vi "MakeInitialOMFJSON.vi"(0 "OMF Container ID":string, 1 "OMF Static Type ID":string, 2 "OMF Static Type Property Names, Formats, and Values":T2(array[cluster]), 3 "OMF Dynamic Type ID":string, 4 "OMF Dynamic Type Property Names and Formats":T1(array[cluster]), 5 "OMF Static Type Instance Name":string) -> (14 "OMF Static Type Message JSON":string, 15 "OMF Dynamic Type Message JSON":string, 16 "OMF Container Message JSON":string, 17 "OMF Static Type Instance Message JSON":string, 18 "OMF Link Message JSON":string)   [LabVIEW 2014]
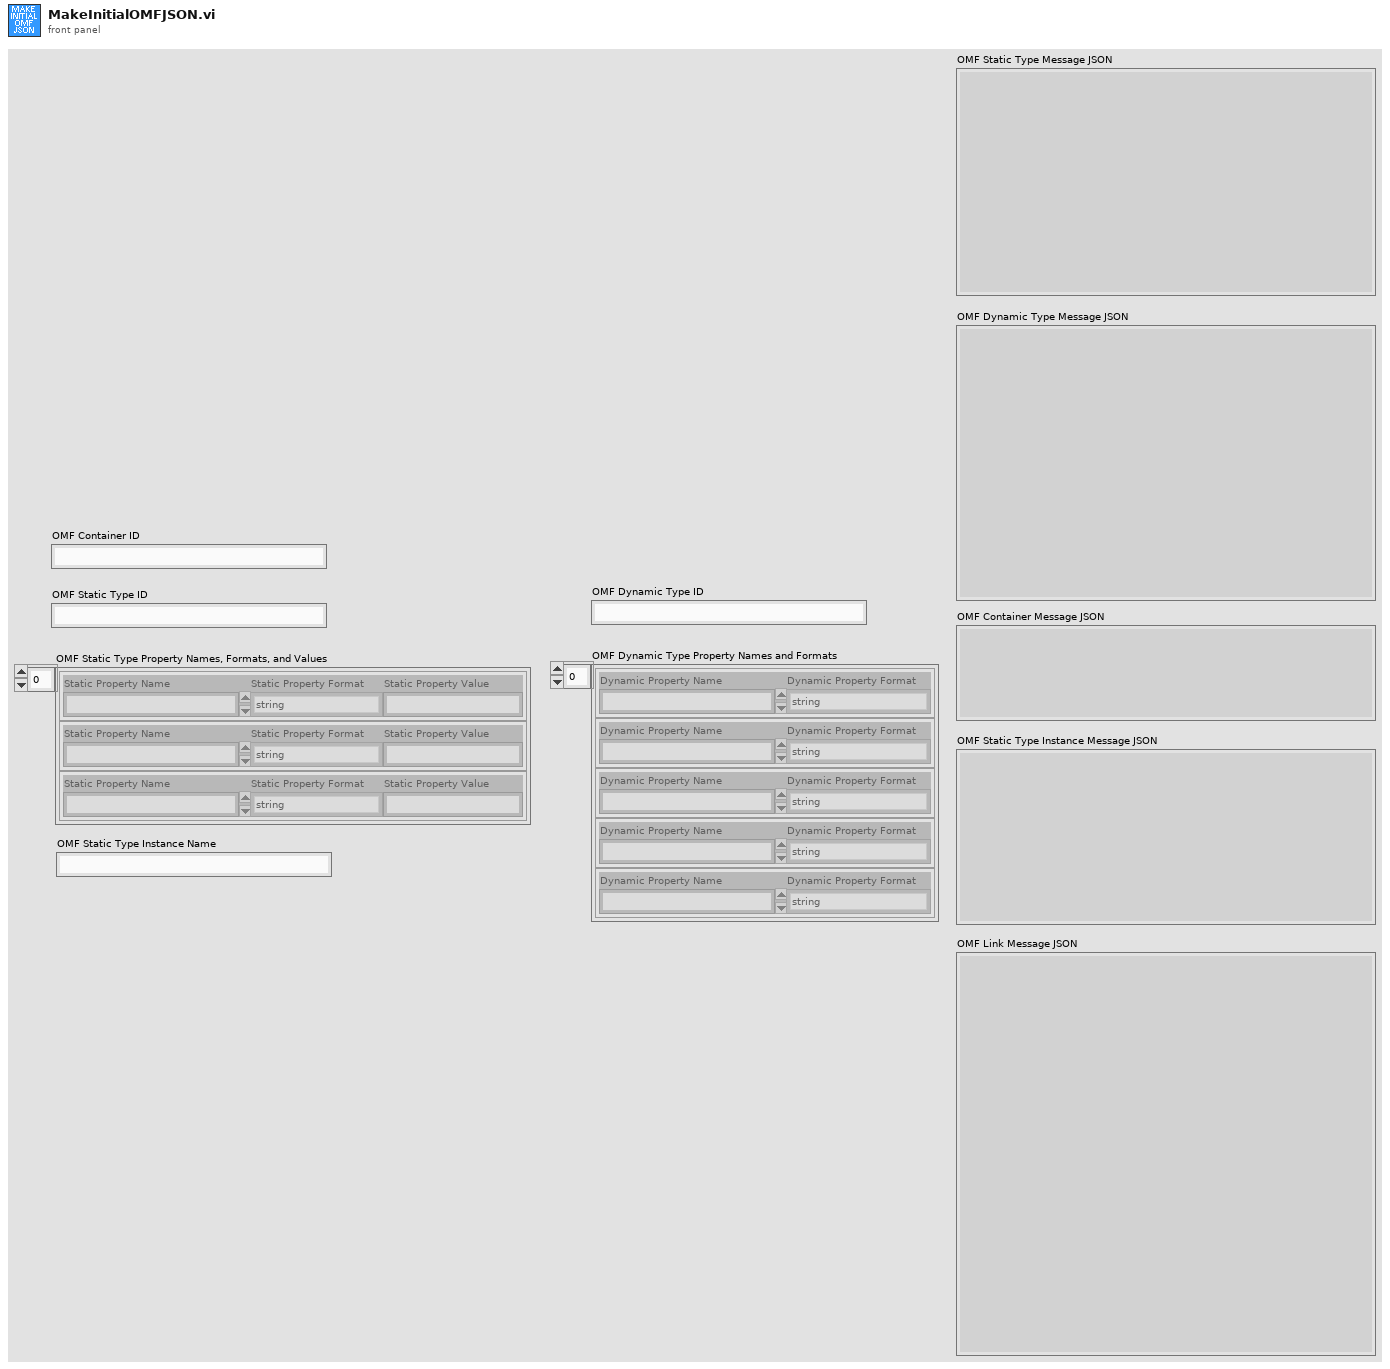
[diagram p1: front panel]
types:
  T1 = cluster{"Dynamic Property Name":string, "Dynamic Property Format":enum16{"string", "number"}}[]
  T2 = cluster{"Static Property Name":string, "Static Property Format":enum16{"string", "number"}, "Static Property Value":string}[]
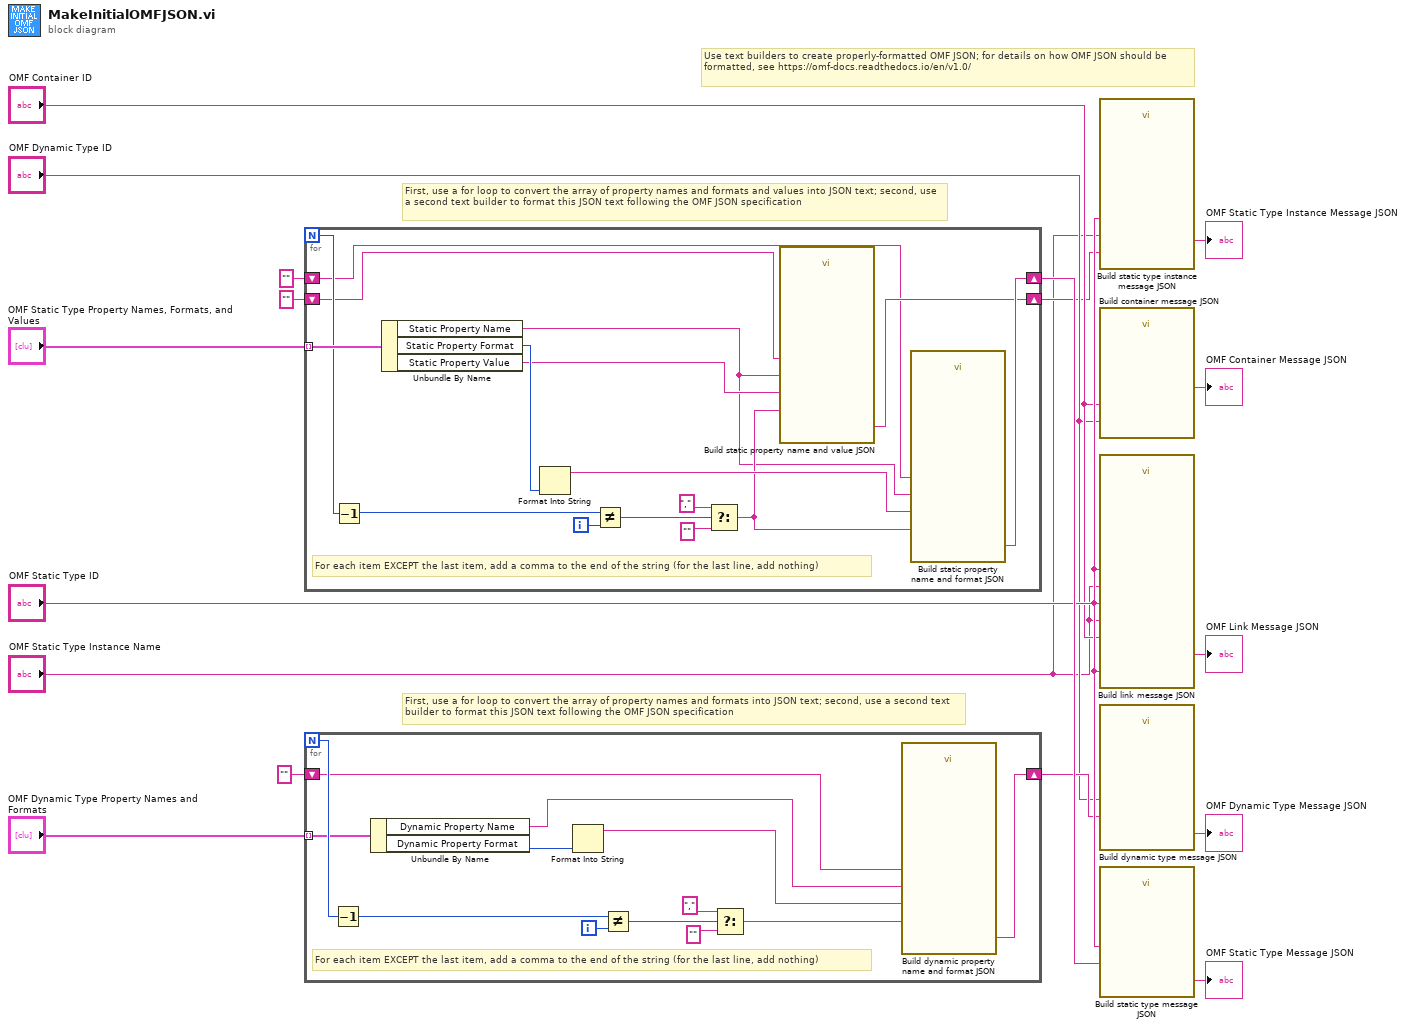
[diagram p0: block diagram]
diagram:
  # "First, use a for loop to convert the array of property names and formats and values into JSON text; second, use a second text builder to format this JSON text following the OMF JSON specification"
  # "First, use a for loop to convert the array of property names and formats into JSON text; second, use a second text builder to format this JSON text following the OMF JSON specification"
  # "Use text builders to create properly-formatted OMF JSON; for details on how OMF JSON should be formatted, see https://omf-docs.readthedocs.io/en/v1.0/"
  n1 = for {
    N -> [w31]
    tunnel: "OMF Static Type Property Names, Formats, and Values" -> [w33] mode=indexing
    shift-right: [w25] -> w14
    shift-left: "" -> [w20]
    shift-right: [w22] -> w3
    shift-left: "" ("Result") -> [w18]
    i -> [w32]
    # "For each item EXCEPT the last item, add a comma to the end of the string (for the last line, add nothing)"
    n2 = Decrement(x=w31) -> (x-1=w30:i32)
    n3 = Unbundle By Name "Unbundle By Name"(w33) -> ("Static Property Name"=w19:string, "Static Property Format"=w26:enum16{"string", "number"}, "Static Property Value"=w21:string)
    n4 = Format Into String "Format Into String"(w26) -> (resulting string=w24:string)  [unwired: 3 in, 1 out]
    n5 = Not Equal?(x=w30, y=w32) -> (x != y?=w29:bool)
    n6 = Select(t="," ("string"), s=w29, f="" ("string")) -> (s? t:f=w23:string)
    n7 = call "Build static property name and value JSON"("End Text"=w23, "Begin Text"=w18, "Property Name"=w19, "Property Value"=w21) -> ("Result"=w22:string)  [unwired: 10 in, 1 out]
    n8 = call "Build static property name and format JSON"("End Text"=w23, "Begin Text"=w20, "Property Name"=w19, "Property Format"=w24) -> ("Result"=w25:string)  [unwired: 10 in, 1 out]
  }
  n9 = for {
    N -> [w45]
    shift-right: [w38] -> w6
    shift-left: "" -> [w36]
    tunnel: "OMF Dynamic Type Property Names and Formats" -> [w41] mode=indexing
    i -> [w46]
    # "For each item EXCEPT the last item, add a comma to the end of the string (for the last line, add nothing)"
    n10 = Decrement(x=w45) -> (x-1=w44:i32)
    n11 = Unbundle By Name "Unbundle By Name"(w41) -> ("Dynamic Property Name"=w35:string, "Dynamic Property Format"=w39:enum16{"string", "number"})
    n12 = Format Into String "Format Into String"(w39) -> (resulting string=w34:string)  [unwired: 3 in, 1 out]
    n13 = Not Equal?(x=w44, y=w46) -> (x != y?=w43:bool)
    n14 = Select(t="," ("string"), s=w43, f="" ("string")) -> (s? t:f=w37:string)
    n15 = call "Build dynamic property name and format JSON"("End Text"=w37, "Begin Text"=w36, "Property Name"=w35, "Property Format"=w34) -> ("Result"=w38:string)  [unwired: 10 in, 1 out]
  }
  n16 = call "Build static type instance message JSON"("OMF Static Type ID"="OMF Static Type ID", "OMF Static Type Instance Name"="OMF Static Type Instance Name", "OMF Static Type Properties and Values"=w3) -> ("Result"=→"OMF Static Type Instance Message JSON":string)  [unwired: 11 in, 1 out]
  n17 = call "Build container message JSON"("OMF Container ID"="OMF Container ID", "OMF Dynamic Type ID"="OMF Dynamic Type ID") -> ("Result"=→"OMF Container Message JSON":string)  [unwired: 12 in, 1 out]
  n18 = call "Build link message JSON"("OMF Static Type ID__"="OMF Static Type ID", "OMF Container ID"="OMF Container ID", "OMF Static Type ID"="OMF Static Type ID", "OMF Static Type ID_"="OMF Static Type ID", "OMF Static Type Instance Name_"="OMF Static Type Instance Name", "OMF Static Type Instance Name__"="OMF Static Type Instance Name") -> ("Result"=→"OMF Link Message JSON":string)  [unwired: 8 in, 1 out]
  n19 = call "Build dynamic type message JSON"("OMF Dynamic Type ID"="OMF Dynamic Type ID", "OMF Dynamic Type Properties JSON"=w6) -> ("Result"=→"OMF Dynamic Type Message JSON":string)  [unwired: 12 in, 1 out]
  n20 = call "Build static type message JSON"("OMF Static Type ID"="OMF Static Type ID", "OMF Static Type Properties JSON"=w14) -> ("Result"=→"OMF Static Type Message JSON":string)  [unwired: 12 in, 1 out]
